vi "write_freq.vi"(8 "error in (no error)":errorcluster, 10 "number":dbl, 11 "VISA Refnum in":refnum<visa-resource-name>) -> (0 "error out":errorcluster, 3 "VISA Refnum out":refnum<visa-resource-name>)   [LabVIEW 2009]
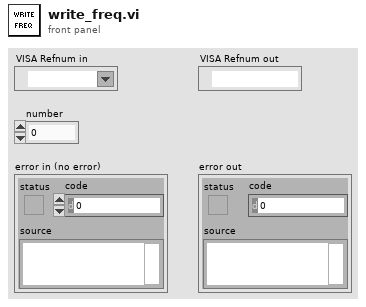
[diagram p1: front panel]
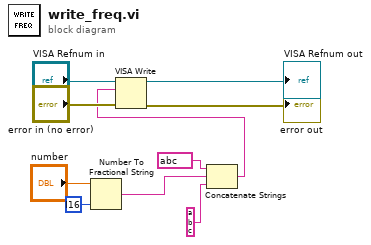
[diagram p0: block diagram]
diagram:
  n1 = Number To Fractional String(number="number", precision (6)=i16 ?) -> (F-format string=w6:string)  [unwired: 2 in]
  n2 = Concatenate Strings(string ? ("write buffer"), w6, string ?) -> (w7:string)
  n3 = VISA Write(VISA resource name="VISA Refnum in", write buffer=w7, error in (no error)="error in (no error)") -> (VISA resource name out=→"VISA Refnum out":refnum<visa-resource-name>, error out=→"error out":errorcluster)  [unwired: 1 out]
